vi "Dequeue.vi"(8 "error in (no error)":errorcluster, 11 "Master in":refnum<class "Master.lvclass">) -> (0 "error out":errorcluster, 2 "State":string, 3 "Master out":refnum<class "Master.lvclass">)   [LabVIEW 2014, in "Master.lvclass"]
uses:
  Master.lvclass
  Master.lvclass/Master.ctl
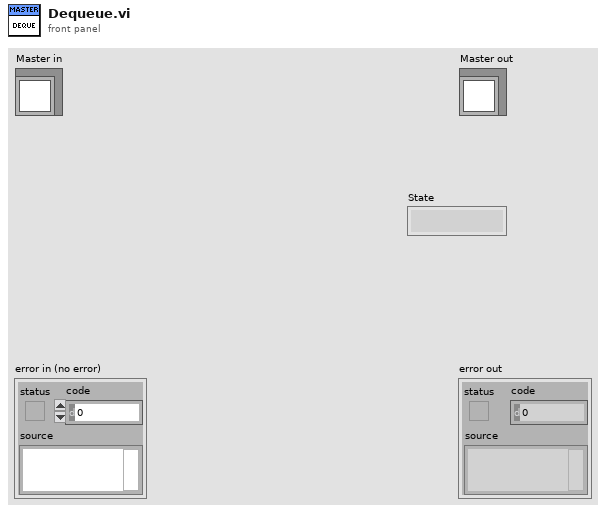
[diagram p1: front panel]
types:
  T1 = typedef "Control Library.lvlib/StateDatas.ctl" = cluster{"State":string, "Data":variant}
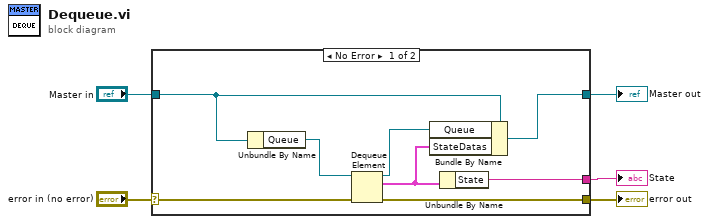
[diagram p0: block diagram]
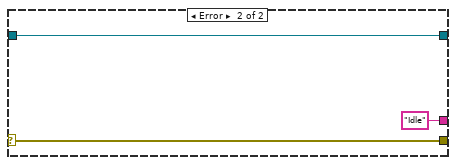
[diagram p2: hidden frame]
diagram:
  n1 = case shown="No Error" "error in (no error)" {
    selector: "error in (no error)" -> [w12 w16]
    tunnel: [w11 w16] -> w4
    tunnel: [w9 w15] -> w2
    tunnel: "Master in" -> [w10 w15]
    tunnel: [w6 "Idle" ("State")] -> w1
    frame No Error {
      n2 = Unbundle By Name(w10) -> ("Queue"=w13:refnum<queue>)
      n3 = Dequeue Element(queue=w13, error in (no error)=w12) -> (queue out=w8:refnum<queue>, element=w7:T1, error out=w11:errorcluster)  [unwired: 1 in, 1 out]
      n4 = Bundle By Name(cluster=w10, "Queue"=w8, "StateDatas"=w7) -> (w9:refnum<class "Master.lvclass">)
      n5 = Unbundle By Name(w7) -> ("State"=w6:string)
    }
    frame Error {
    }
  }
  "error out" <- w4
  "Master out" <- w2
  "State" <- w1
